vi "GenerateSelectionList.vi"(11 "ref通道选择":refnum<vi>) -> ()   [LabVIEW 2018, in "DataDisplay.lvlib"]
uses:
  DataDisplay.lvlib
  DD_Parameter.vi
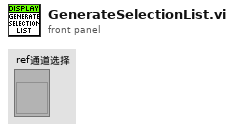
[diagram p1: front panel]
types:
  T1 = typedef "DataDisplay.lvlib/DD_ChannelInfo.ctl" = cluster{"名称":string, "单位":string, "数据类型":enum16{"Real", "Int"}, "趋势线":enum16{"N/A", "X", "Y"}}
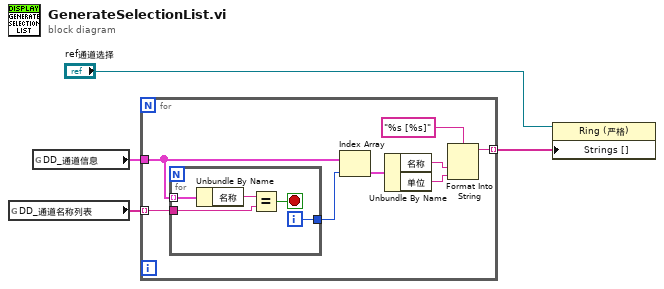
[diagram p0: block diagram]
diagram:
  n1 = global read "DD_Parameter.vi" "DD_通道名称列表"() -> (w1:string[])
  n2 = global read "DD_Parameter.vi" "DD_通道信息"() -> (w2:T1[])
  n3 = for {
    tunnel: w1 -> [w12] mode=indexing
    tunnel: w2 -> [w8]
    tunnel: [w5] -> w3 mode=indexing
    n4 = for {
      tunnel: w8 -> [w17] mode=indexing
      tunnel: w12 -> [w15]
      tunnel: [w13] -> w7
      i -> [w13]
      stop <- w14 stop-if-true
      n5 = Unbundle By Name(w17) -> ("名称"=w16:string)
      n6 = Equal?(x=w16, y=w15) -> (x = y?=w14:bool)
    }
    n7 = Index Array(array=w8, index=w7) -> (element=w6:T1)
    n8 = Unbundle By Name(w6) -> ("名称"=w10:string, "单位"=w11:string)
    n9 = Format Into String(format string="%s [%s]" ("格式字符串"), w10, w11) -> (resulting string=w5:string)  [unwired: 2 in, 1 out]
  }
  n10 = property class="Ring (严格)"(reference="ref通道选择", "Strings []"=w3) -> ()  [unwired: 1 in, 2 out]
